vi "switch_subplot.vi"() -> ()   [LabVIEW 2018]
uses:
  Settings/Settings.ctl
  Acquisition/Hardware Configuration.ctl
  Acquisition/Signal Type.ctl
  Logging/Logging Configuration.ctl
  Logging/Logging.lvlib
  Acquisition/Acquisition.lvlib
  Settings/Settings.lvlib
panel:
  out "配置输出":T1 {"串口通信UI"."Format" items=["标准帧", "扩展帧"]; "串口通信UI"."Type" items=["数据帧", "远程帧"]; "串口通信UI"."ID" format="0x%x"; "串口通信UI"."Fliter" items=["接收所有类型"=1, "只接收标准帧"=2, "只接收扩展帧"=3]; "串口通信UI"."kBaudRate" items=["5k bps"=1, "10k bps"=2, "20k bps"=3, "40k bps"=4, "50k bps"=5, "80k bps"=6, "100k bps"=7, "125k bps"=8, "200k bps"=9, "250k bps"=10, "400k bps"=11, "500k bps"=12, "666k bps"=13, "800k bps"=14, "1000k bps"=15, "33.33k bps"=16, "66.66k bps"=17, "83.33k bps"=18]; "串口通信UI"."Mode" items=["正常工作", "仅侦听模式", "自测模式（环回）"]; "串口通信UI"."InitFlag" items=["使用界面设置参数"=1]; "串口通信UI"."AccMask" format="%08x"; "串口通信UI"."AccCode" format="%08x"; "串口通信UI"."Channel" items=["通道1", "通道2"]; "串口通信UI"."DevType" items=["USB-CAN"=3, "USB-CAN2"=4]; "安全报警UI"."操作 8" items=["产生报警信息（不发声），等待手动操作", "产生报警信息（发声），等待手动操作", "产生报警信息（不发声），自动刹车", "产生报警信息（发声），自动刹车", "产生报警信息（不发声），立即自动断电，开启泄放电阻", "产生报警信息（发声），立即自动断电，开启泄放电阻"]; "安全报警UI"."操作 7" items=["产生报警信息（不发声），等待手动操作", "产生报警信息（发声），等待手动操作", "产生报警信息（不发声），自动刹车", "产生报警信息（发声），自动刹车", "产生报警信息（不发声），立即自动断电，开启泄放电阻", "产生报警信息（发声），立即自动断电，开启泄放电阻"]; "安全报警UI"."操作 6" items=["产生报警信息（不发声），等待手动操作", "产生报警信息（发声），等待手动操作", "产生报警信息（不发声），自动刹车", "产生报警信息（发声），自动刹车", "产生报警信息（不发声），立即自动断电，开启泄放电阻", "产生报警信息（发声），立即自动断电，开启泄放电阻"]; "安全报警UI"."操作 5" items=["产生报警信息（不发声），等待手动操作", "产生报警信息（发声），等待手动操作", "产生报警信息（不发声），自动刹车", "产生报警信息（发声），自动刹车", "产生报警信息（不发声），立即自动断电，开启泄放电阻", "产生报警信息（发声），立即自动断电，开启泄放电阻"]; "安全报警UI"."操作 4" items=["产生报警信息（不发声），等待手动操作", "产生报警信息（发声），等待手动操作", "产生报警信息（不发声），自动刹车", "产生报警信息（发声），自动刹车", "产生报警信息（不发声），立即自动断电，开启泄放电阻", "产生报警信息（发声），立即自动断电，开启泄放电阻"]; "安全报警UI"."操作 3" items=["产生报警信息（不发声），等待手动操作", "产生报警信息（发声），等待手动操作", "产生报警信息（不发声），自动刹车", "产生报警信息（发声），自动刹车", "产生报警信息（不发声），立即自动断电，开启泄放电阻", "产生报警信息（发声），立即自动断电，开启泄放电阻"]; "安全报警UI"."操作 2" items=["产生报警信息（不发声），等待手动操作", "产生报警信息（发声），等待手动操作", "产生报警信息（不发声），自动刹车", "产生报警信息（发声），自动刹车", "产生报警信息（不发声），立即自动断电，开启泄放电阻", "产生报警信息（发声），立即自动断电，开启泄放电阻"]; "安全报警UI"."操作" items=["产生报警信息（不发声），等待手动操作", "产生报警信息（发声），等待手动操作", "产生报警信息（不发声），自动刹车", "产生报警信息（发声），自动刹车", "产生报警信息（不发声），立即自动断电，开启泄放电阻", "产生报警信息（发声），立即自动断电，开启泄放电阻"]}
  in  "配置":T1 {"串口通信UI"."Format" items=["标准帧", "扩展帧"]; "串口通信UI"."Type" items=["数据帧", "远程帧"]; "串口通信UI"."ID" format="0x%x"; "串口通信UI"."Fliter" items=["接收所有类型"=1, "只接收标准帧"=2, "只接收扩展帧"=3]; "串口通信UI"."kBaudRate" items=["5k bps"=1, "10k bps"=2, "20k bps"=3, "40k bps"=4, "50k bps"=5, "80k bps"=6, "100k bps"=7, "125k bps"=8, "200k bps"=9, "250k bps"=10, "400k bps"=11, "500k bps"=12, "666k bps"=13, "800k bps"=14, "1000k bps"=15, "33.33k bps"=16, "66.66k bps"=17, "83.33k bps"=18]; "串口通信UI"."Mode" items=["正常工作", "仅侦听模式", "自测模式（环回）"]; "串口通信UI"."InitFlag" items=["使用界面设置参数"=1]; "串口通信UI"."AccMask" format="%08x"; "串口通信UI"."AccCode" format="%08x"; "串口通信UI"."Channel" items=["通道1", "通道2"]; "串口通信UI"."DevType" items=["USB-CAN"=3, "USB-CAN2"=4]; "安全报警UI"."操作 8" items=["产生报警信息（不发声），等待手动操作", "产生报警信息（发声），等待手动操作", "产生报警信息（不发声），自动刹车", "产生报警信息（发声），自动刹车", "产生报警信息（不发声），立即自动断电，开启泄放电阻", "产生报警信息（发声），立即自动断电，开启泄放电阻"]; "安全报警UI"."操作 7" items=["产生报警信息（不发声），等待手动操作", "产生报警信息（发声），等待手动操作", "产生报警信息（不发声），自动刹车", "产生报警信息（发声），自动刹车", "产生报警信息（不发声），立即自动断电，开启泄放电阻", "产生报警信息（发声），立即自动断电，开启泄放电阻"]; "安全报警UI"."操作 6" items=["产生报警信息（不发声），等待手动操作", "产生报警信息（发声），等待手动操作", "产生报警信息（不发声），自动刹车", "产生报警信息（发声），自动刹车", "产生报警信息（不发声），立即自动断电，开启泄放电阻", "产生报警信息（发声），立即自动断电，开启泄放电阻"]; "安全报警UI"."操作 5" items=["产生报警信息（不发声），等待手动操作", "产生报警信息（发声），等待手动操作", "产生报警信息（不发声），自动刹车", "产生报警信息（发声），自动刹车", "产生报警信息（不发声），立即自动断电，开启泄放电阻", "产生报警信息（发声），立即自动断电，开启泄放电阻"]; "安全报警UI"."操作 4" items=["产生报警信息（不发声），等待手动操作", "产生报警信息（发声），等待手动操作", "产生报警信息（不发声），自动刹车", "产生报警信息（发声），自动刹车", "产生报警信息（不发声），立即自动断电，开启泄放电阻", "产生报警信息（发声），立即自动断电，开启泄放电阻"]; "安全报警UI"."操作 3" items=["产生报警信息（不发声），等待手动操作", "产生报警信息（发声），等待手动操作", "产生报警信息（不发声），自动刹车", "产生报警信息（发声），自动刹车", "产生报警信息（不发声），立即自动断电，开启泄放电阻", "产生报警信息（发声），立即自动断电，开启泄放电阻"]; "安全报警UI"."操作 2" items=["产生报警信息（不发声），等待手动操作", "产生报警信息（发声），等待手动操作", "产生报警信息（不发声），自动刹车", "产生报警信息（发声），自动刹车", "产生报警信息（不发声），立即自动断电，开启泄放电阻", "产生报警信息（发声），立即自动断电，开启泄放电阻"]; "安全报警UI"."操作" items=["产生报警信息（不发声），等待手动操作", "产生报警信息（发声），等待手动操作", "产生报警信息（不发声），自动刹车", "产生报警信息（发声），自动刹车", "产生报警信息（不发声），立即自动断电，开启泄放电阻", "产生报警信息（发声），立即自动断电，开启泄放电阻"]}
  in  "簇":T23
  # "参数配置文件"
  # "输入数据文件"
  # "加载电机"
  # "负载电机"
  # "注：每次运行实验时销毁现有所有图像"
  # "参数配置文件"
  # "输入数据文件"
  # "加载电机"
  # "负载电机"
  # "注：每次运行实验时销毁现有所有图像"
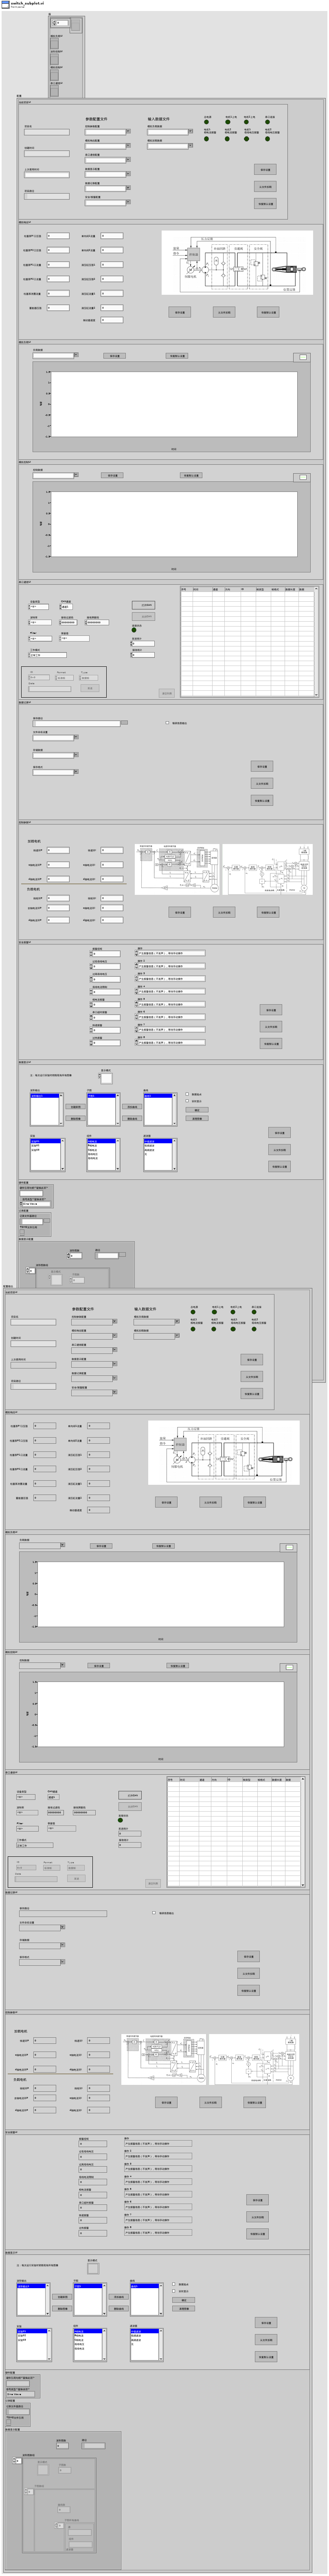
[diagram p1: front panel]
types:
  T1 = typedef "Settings.lvlib/Settings.ctl" = cluster{"当前项目UI":T2, "模拟响应UI":T3, "模拟负载UI":T4, "模拟控制UI":T5, "串口通信UI":T6, "数据记录UI":T12, "控制参数UI":T13, "安全报警UI":T14, "数据显示UI":T15, "硬件配置":T16, "记录配置":T18, "数据显示配置":T19}
  T2 = typedef "控件 5.ctl" = cluster{"控制参数配置":string, "模拟响应配置":string, "串口通信配置":string, "数据显示配置":string, "数据记录配置":string, "安全/报警配置":string, "模拟负载数据":string, "模拟加载数据":string, "总电源":bool, "电机1上电":bool, "电机2上电":bool, "串口连接":bool, "电机1\n相电流报警":bool, "电机2\n相电流报警":bool, "电机1\n母线电压报警":bool, "电机2\n母线电压报警":bool, "保存设置":bool, "从文件加载":bool, "恢复默认设置":bool, "路径":path, "项目路径":path, "项目名":string, "创建时间":string, "上次使用时间":string}
  T3 = typedef "模拟响应UI.ctl" = cluster{"柱塞泵P!口压强":dbl, "柱塞泵P2口压强":dbl, "柱塞泵P1口流量":dbl, "柱塞泵P2口流量":dbl, "柱塞泵泄露流量":dbl, "蓄能器压强":dbl, "单向阀1流量":dbl, "单向阀2流量":dbl, "液压缸压强1":dbl, "液压缸压强2":dbl, "液压缸流量1":dbl, "液压缸流量2":dbl, "做动器速度":dbl, "保存设置":bool, "从文件加载":bool, "恢复默认设置":bool, "路径":path}
  T4 = typedef "控件 9.ctl" = cluster{"负载数据":string, "负载数据 2":waveform(dbl)[], "保存设置":bool, "恢复默认设置":bool}
  T5 = typedef "控件 7.ctl" = cluster{"控制数据":string, "负载数据 2":waveform(dbl)[], "保存设置":bool, "恢复默认设置":bool}
  T6 = typedef "控件 6.ctl" = cluster{"DevType":T7, "Channel":T8, "AccCode":u32, "AccMask":u32, "InitFlag":T9, "Mode":T10, "kBaudRate":u8, "Fliter":T11, "Open":bool, "Close":bool, "连接状态":bool, "SendCnt":u32, "RecvCnt":u32, "Send":bool, "ID":u32, "Data":string, "Type":u8, "Format":u8, "Clear":bool, "list":i32, "路径":path}
  T7 = typedef "ControlCAN.lvlib/DevType.ctl" = u32
  T8 = typedef "ControlCAN.lvlib/CAN Channel.ctl" = u32
  T9 = typedef "ControlCAN.lvlib/InitFlag.ctl" = u32
  T10 = typedef "ControlCAN.lvlib/Mode.ctl" = u8
  T11 = typedef "ControlCAN.lvlib/Fliter.ctl" = u8
  T12 = typedef "控件 3.ctl" = cluster{"保存路径":path, "文件命名设置":string, "存储数据":string, "保存格式":string, "复选框":bool, "保存设置":bool, "从文件加载":bool, "恢复默认设置":bool, "路径":path}
  T13 = typedef "控件 1.ctl" = cluster{"d轴电流环P":dbl, "转速环P":dbl, "q轴电流环P":dbl, "d轴电流环P":dbl, "转矩环P":dbl, "去轴电流环P":dbl, "转速环I":dbl, "q轴电流环I":dbl, "d轴电流环I":dbl, "转矩环I":dbl, "q轴电流环I":dbl, "d轴电流环I":dbl, "保存设置":bool, "从文件加载":bool, "恢复默认设置":bool, "路径":path}
  T14 = typedef "控件 4.ctl" = cluster{"报警扭矩":dbl, "过低母线电压":dbl, "过高母线电压":dbl, "母线电流限制":dbl, "相电流报警":dbl, "串口超时报警":dbl, "转速报警":dbl, "过热报警":dbl, "操作":u16, "操作 2":u16, "操作 3":u16, "操作 4":u16, "操作 5":u16, "操作 6":u16, "操作 7":u16, "操作 8":u16, "保存设置":bool, "从文件加载":bool, "恢复默认设置":bool, "路径":path}
  T15 = typedef "控件 2.ctl" = cluster{"保存设置":bool, "从文件加载":bool, "恢复默认设置":bool, "实验":i32, "波形输出":i32, "组件":i32, "曲线":i32, "滤波器":i32, "删除曲线":bool, "清理图像":bool, "添加曲线":bool, "数据选点":bool, "确定按钮":bool, "实时显示":bool, "子图":i32, "显示模式":u16, "路径":path, "删除图像":bool, "创建新图":bool}
  T16 = typedef "Acquisition.lvlib/Hardware Configuration.ctl" = cluster{"硬件引用句柄<替换此项>":string, "信号类型<替换该项>":T17}
  T17 = typedef "Acquisition.lvlib/Signal Type.ctl" = enum16{"Sine Wave", "Square with Noise"}
  T18 = typedef "Logging.lvlib/Logging Configuration.ctl" = cluster{"记录文件基路径":path, "TDMS文件引用":refnum<k34>}
  T19 = typedef "波形图簇.ctl" = cluster{"波形图数":u32, "波形图数组":T20[], "路径":path}
  T20 = typedef "波形图.ctl" = cluster{"显示模式":u16, "子图数":u32, "子图数组":T21[]}
  T21 = typedef "子图.ctl" = cluster{"子图所有曲线":T22[], "曲线数":u32}
  T22 = typedef "曲线簇.ctl" = cluster{"源":string, "组件":string, "滤波器":string}
  T23 = typedef "引用簇.ctl" = cluster{"数组":refnum<vi>[], "模拟负载UI":refnum<vi>, "波形控制UI":refnum<vi>, "模拟控制UI":refnum<vi>, "串口通信UI":refnum<vi>, "当前项目UI":refnum<vi>, "安全报警UI":refnum<vi>, "数据记录UI":refnum<vi>, "数据显示UI":refnum<vi>, "控制参数UI":refnum<vi>, "模拟响应UI":refnum<vi>, "主选项卡UI":refnum<vi>, "项目管理UI":refnum<vi>, "开始":refnum<vi>, "设置":refnum<vi>, "停止":refnum<vi>, "退出":refnum<vi>}
  T24 = enum8{"Enabled", "Disabled", "Disabled and Grayed Out"}
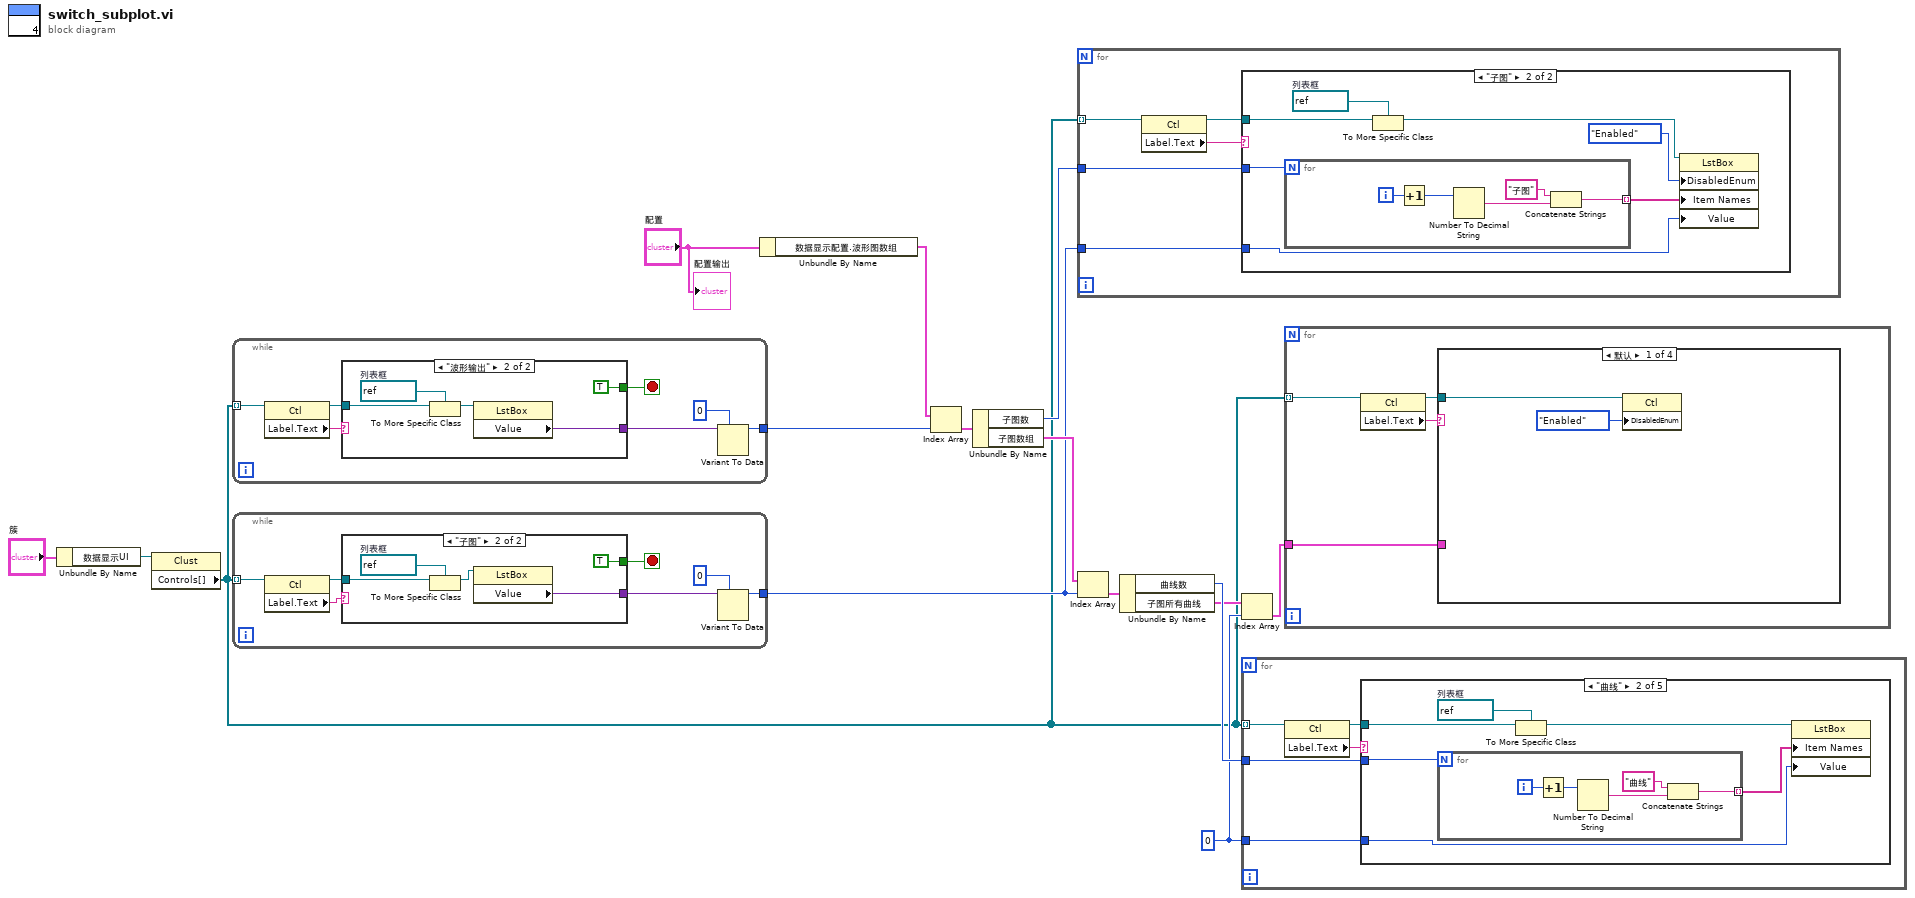
[diagram p0: block diagram]
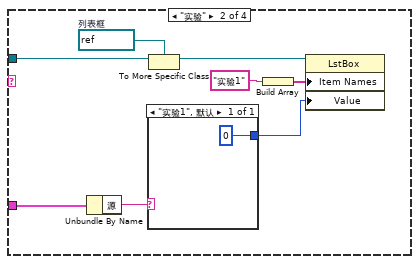
[diagram p2: hidden frame]
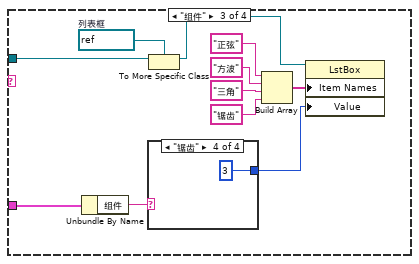
[diagram p3: hidden frame]
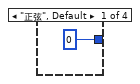
[diagram p4: hidden frame]
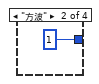
[diagram p5: hidden frame]
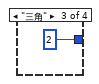
[diagram p6: hidden frame]
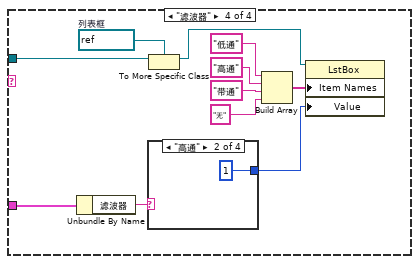
[diagram p7: hidden frame]
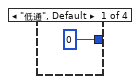
[diagram p8: hidden frame]
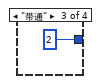
[diagram p9: hidden frame]
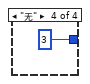
[diagram p10: hidden frame]
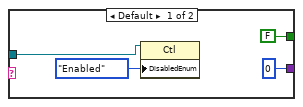
[diagram p11: hidden frame]
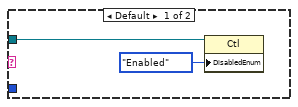
[diagram p12: hidden frame]
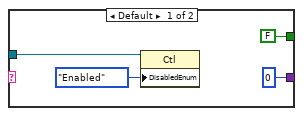
[diagram p13: hidden frame]
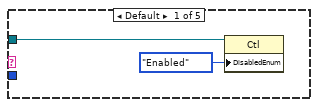
[diagram p14: hidden frame]
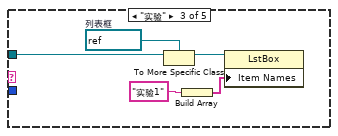
[diagram p15: hidden frame]
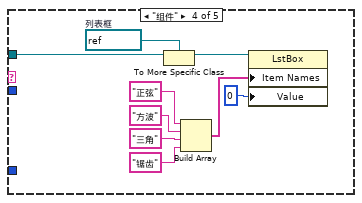
[diagram p16: hidden frame]
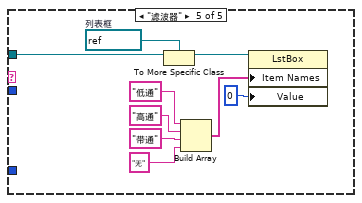
[diagram p17: hidden frame]
diagram:
  w3 = 0
  n1 = Unbundle By Name("簇") -> ("数据显示UI"=w14:refnum<vi>)
  n2 = property class="Clust"(reference=w14) -> ("Controls[]"=w2:refnum<vi>[])  [unwired: 1 in, 2 out]
  n3 = while {
    tunnel: w2 -> [w22] mode=indexing
    tunnel: [w17] -> w10
    stop <- w19 stop-if-true
    n4 = property class="Ctl"(reference=w22) -> (reference out=w20:refnum<vi>, "Label.Text"=w21:string)  [unwired: 1 in, 1 out]
    n5 = case shown="\"波形输出\"" w21 {
      tunnel: w20 -> [w26 w31]
      tunnel: [0 w27] -> w18
      tunnel: [FALSE TRUE] -> w19
      frame Default {
        n6 = property class="Ctl"(reference=w26, "DisabledEnum"=T24."Enabled" ("禁用")) -> ()  [unwired: 1 in, 2 out]
      }
      frame "波形输出" {
        w30 = refnum<vi> refnum  # 列表框
        n7 = To More Specific Class(target class=w30, reference=w31) -> (specific class reference=w29:refnum<vi>)  [unwired: 1 in, 1 out]
        n8 = property class="LstBox"(reference=w29) -> ("Value"=w27:variant)  [unwired: 1 in, 2 out]
      }
    }
    n9 = Variant To Data(type=0, Variant=w18) -> (data=w17:i32)  [unwired: 1 in, 1 out]
  }
  n10 = while {
    tunnel: w2 -> [w38] mode=indexing
    tunnel: [w33] -> w5
    stop <- w35 stop-if-true
    n11 = property class="Ctl"(reference=w38) -> (reference out=w36:refnum<vi>, "Label.Text"=w37:string)  [unwired: 1 in, 1 out]
    n12 = case shown="\"子图\"" w37 {
      tunnel: w36 -> [w42 w47]
      tunnel: [0 w43] -> w34
      tunnel: [FALSE TRUE] -> w35
      frame Default {
        n13 = property class="Ctl"(reference=w42, "DisabledEnum"=T24."Enabled" ("禁用")) -> ()  [unwired: 1 in, 2 out]
      }
      frame "子图" {
        w46 = refnum<vi> refnum  # 列表框
        n14 = To More Specific Class(target class=w46, reference=w47) -> (specific class reference=w45:refnum<vi>)  [unwired: 1 in, 1 out]
        n15 = property class="LstBox"(reference=w45) -> ("Value"=w43:variant)  [unwired: 1 in, 2 out]
      }
    }
    n16 = Variant To Data(type=0, Variant=w34) -> (data=w33:i32)  [unwired: 1 in, 1 out]
  }
  n17 = Unbundle By Name("配置") -> ("数据显示配置.波形图数组"=w11:T20[])
  n18 = Index Array(array=w11, index=w10) -> (element=w12:T20)
  n19 = Unbundle By Name(w12) -> ("子图数"=w8:u32, "子图数组"=w7:T21[])
  n20 = for {
    tunnel: w2 -> [w50] mode=indexing
    tunnel: w8 -> [w49]
    tunnel: w5 -> [w48]
    n21 = property class="Ctl"(reference=w50) -> (reference out=w51:refnum<vi>, "Label.Text"=w52:string)  [unwired: 1 in, 1 out]
    n22 = case shown="\"子图\"" w52 {
      tunnel: w51 -> [w54 w60]
      tunnel: w49 -> [_ w56]
      tunnel: w48 -> [_ w55]
      frame Default {
        n23 = property class="Ctl"(reference=w54, "DisabledEnum"=T24."Enabled" ("禁用")) -> ()  [unwired: 1 in, 2 out]
      }
      frame "子图" {
        w59 = refnum<vi> refnum  # 列表框
        n24 = for {
          N: w56 -> [_]
          tunnel: [w64] -> w57 mode=indexing
          i -> [w66]
          n25 = Increment(x=w66) -> (x+1=w62:i32)
          n26 = Number To Decimal String(number=w62) -> (decimal integer string=w63:string)  [unwired: 1 in]
          n27 = Concatenate Strings("子图", w63) -> (w64:string)
        }
        n28 = To More Specific Class(target class=w59, reference=w60) -> (specific class reference=w58:refnum<vi>)  [unwired: 1 in, 1 out]
        n29 = property class="LstBox"(reference=w58, "DisabledEnum"=T24."Enabled" ("禁用"), "Item Names"=w57, "Value"=w55) -> ()  [unwired: 1 in, 2 out]
      }
    }
  }
  n30 = Index Array(array=w7, index=w5) -> (element=w6:T21)
  n31 = Unbundle By Name(w6) -> ("曲线数"=w13:u32, "子图所有曲线"=w4:T22[])
  n32 = Index Array(array=w4, index=w3) -> (element=w1:T22)
  n33 = for {
    tunnel: w2 -> [w71] mode=indexing
    tunnel: w13 -> [w68]
    tunnel: w3 -> [w67]
    n34 = property class="Ctl"(reference=w71) -> (reference out=w69:refnum<vi>, "Label.Text"=w70:string)  [unwired: 1 in, 1 out]
    n35 = case shown="\"曲线\"" w70 {
      tunnel: w69 -> [w73 w79 w89 w98 w107]
      tunnel: w68 -> [_ w76 _ _ _]
      tunnel: w67 -> [_ w74 _ _ _]
      frame Default {
        n36 = property class="Ctl"(reference=w73, "DisabledEnum"=T24."Enabled" ("禁用")) -> ()  [unwired: 1 in, 2 out]
      }
      frame "曲线" {
        w78 = refnum<vi> refnum  # 列表框
        n37 = for {
          N: w76 -> [_]
          tunnel: [w80] -> w75 mode=indexing
          i -> [w84]
          n38 = Increment(x=w84) -> (x+1=w83:i32)
          n39 = Number To Decimal String(number=w83) -> (decimal integer string=w81:string)  [unwired: 1 in]
          n40 = Concatenate Strings("曲线", w81) -> (w80:string)
        }
        n41 = To More Specific Class(target class=w78, reference=w79) -> (specific class reference=w77:refnum<vi>)  [unwired: 1 in, 1 out]
        n42 = property class="LstBox"(reference=w77, "Item Names"=w75, "Value"=w74) -> ()  [unwired: 1 in, 2 out]
      }
      frame "实验" {
        w88 = refnum<vi> refnum  # 列表框
        n43 = To More Specific Class(target class=w88, reference=w89) -> (specific class reference=w87:refnum<vi>)  [unwired: 1 in, 1 out]
        n44 = Build Array("实验1") -> (w86:string[])
        n45 = property class="LstBox"(reference=w87, "Item Names"=w86) -> ()  [unwired: 1 in, 2 out]
      }
      frame "组件" {
        w97 = refnum<vi> refnum  # 列表框
        n46 = To More Specific Class(target class=w97, reference=w98) -> (specific class reference=w96:refnum<vi>)  [unwired: 1 in, 1 out]
        n47 = Build Array("正弦", "方波", "三角", "锯齿") -> (w95:string[])
        n48 = property class="LstBox"(reference=w96, "Item Names"=w95, "Value"=0) -> ()  [unwired: 1 in, 2 out]
      }
      frame "滤波器" {
        w106 = refnum<vi> refnum  # 列表框
        n49 = To More Specific Class(target class=w106, reference=w107) -> (specific class reference=w105:refnum<vi>)  [unwired: 1 in, 1 out]
        n50 = Build Array("低通", "高通", "带通", "无") -> (w104:string[])
        n51 = property class="LstBox"(reference=w105, "Item Names"=w104, "Value"=0) -> ()  [unwired: 1 in, 2 out]
      }
    }
  }
  n52 = for {
    tunnel: w2 -> [w111] mode=indexing
    tunnel: w1 -> [w108]
    n53 = property class="Ctl"(reference=w111) -> (reference out=w109:refnum<vi>, "Label.Text"=w110:string)  [unwired: 1 in, 1 out]
    n54 = case shown="默认" w110 {
      tunnel: w109 -> [w113 w121 w133 w148]
      tunnel: w108 -> [_ w115 w125 w139]
      frame Default {
        n55 = property class="Ctl"(reference=w113, "DisabledEnum"=T24."Enabled" ("禁用")) -> ()  [unwired: 1 in, 2 out]
      }
      frame "实验" {
        w120 = refnum<vi> refnum  # 列表框
        n56 = Unbundle By Name(w115) -> ("源"=w116:string)
        n57 = case shown="\"实验1\", 默认" w116 {
          tunnel: [0] -> w114
          frame "实验1", Default {
          }
        }
        n58 = To More Specific Class(target class=w120, reference=w121) -> (specific class reference=w119:refnum<vi>)  [unwired: 1 in, 1 out]
        n59 = Build Array("实验1") -> (w118:string[])
        n60 = property class="LstBox"(reference=w119, "Item Names"=w118, "Value"=w114) -> ()  [unwired: 1 in, 2 out]
      }
      frame "组件" {
        w132 = refnum<vi> refnum  # 列表框
        n61 = Unbundle By Name(w125) -> ("组件"=w124:string)
        n62 = case shown="\"锯齿\"" w124 {
          tunnel: [0 1 2 3] -> w123
          frame "正弦", Default {
          }
          frame "方波" {
          }
          frame "三角" {
          }
          frame "锯齿" {
          }
        }
        n63 = To More Specific Class(target class=w132, reference=w133) -> (specific class reference=w131:refnum<vi>)  [unwired: 1 in, 1 out]
        n64 = Build Array("正弦", "方波", "三角", "锯齿") -> (w130:string[])
        n65 = property class="LstBox"(reference=w131, "Item Names"=w130, "Value"=w123) -> ()  [unwired: 1 in, 2 out]
      }
      frame "滤波器" {
        w147 = refnum<vi> refnum  # 列表框
        n66 = Unbundle By Name(w139) -> ("滤波器"=w140:string)
        n67 = case shown="\"高通\"" w140 {
          tunnel: [0 1 2 3] -> w138
          frame "低通", Default {
          }
          frame "高通" {
          }
          frame "带通" {
          }
          frame "无" {
          }
        }
        n68 = To More Specific Class(target class=w147, reference=w148) -> (specific class reference=w146:refnum<vi>)  [unwired: 1 in, 1 out]
        n69 = Build Array("低通", "高通", "带通", "无") -> (w145:string[])
        n70 = property class="LstBox"(reference=w146, "Item Names"=w145, "Value"=w138) -> ()  [unwired: 1 in, 2 out]
      }
    }
  }
  "配置输出" <- "配置"
